vi "repeat cycle_exponential down.vi"(8 "error in (no error)":errorcluster caption="에러 입력(에러 없음)", 10 "waveform in":waveform(dbl), 11 "Waveform Obj 입력":refnum<class "Waveform Gen.lvclass">) -> (0 "error out":errorcluster caption="에러 출력", 2 "waveform out":waveform(dbl), 3 "Waveform Obj 출력":refnum<class "Waveform Gen.lvclass">)   [LabVIEW 2020, in "Waveform Gen.lvclass"]
uses:
  Waveform Gen.lvclass
  Waveform Gen.lvclass/Waveform Gen.ctl
  Accessors/Read cycle.vi
  <vilib>/Waveform/WDTOps.llb/WDT Append Waveforms DBL.vi
  <vilib>/Waveform/WDTOps.llb/WDT Number of Waveform Samples DBL.vi
  <vilib>/Waveform/WDTOps.llb/WDT Get Waveform Subset DBL.vi
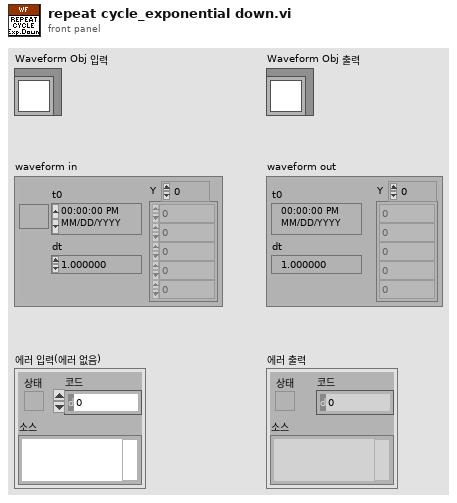
[diagram p1: front panel]
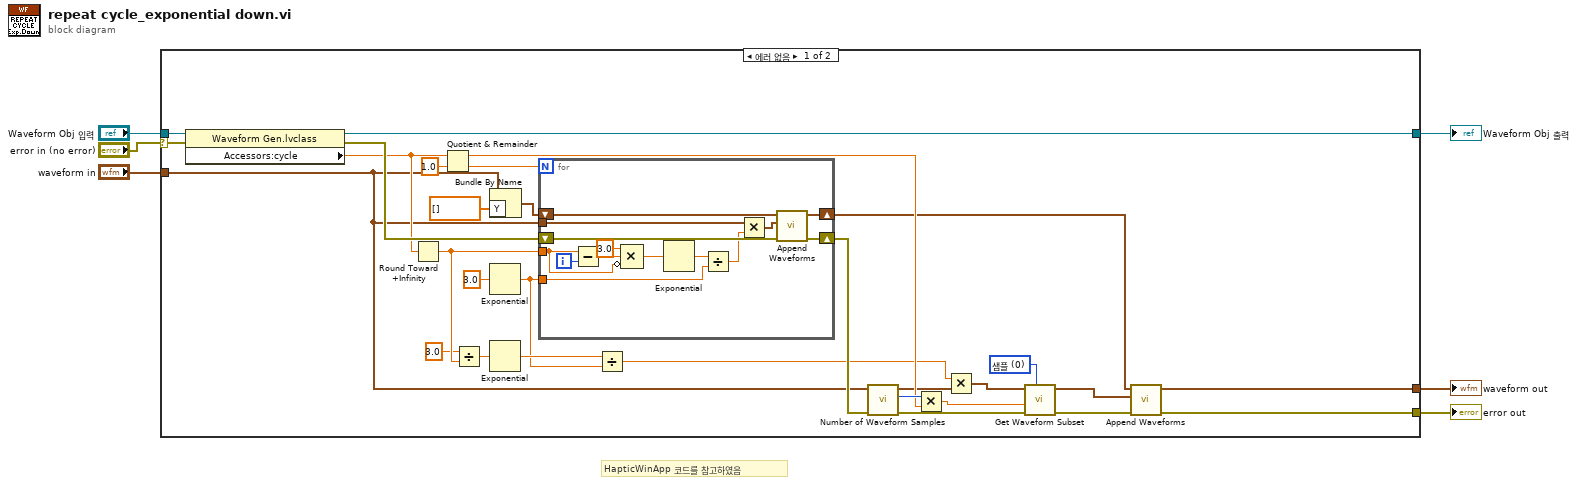
[diagram p0: block diagram]
diagram:
  # "HapticWinApp 코드를 참고하였음"
  n1 = case shown="에러 없음" "error in (no error)" {
    selector: "error in (no error)" -> [w34 w52]
    tunnel: [w8 w52] -> w3
    tunnel: "Waveform Obj 입력" -> [w36 w51]
    tunnel: [w9 w51] -> w4
    tunnel: "waveform in" -> [w10 _]
    tunnel: [w7 _] -> w1
    frame No Error {
      w23 = u16 0 items=["샘플", "상대 시간"] ("start/duration format")
      n2 = property class="Waveform Gen.lvclass"(reference=w36, error in=w34) -> (reference out=w9:refnum<class "Waveform Gen.lvclass">, error out=w27:errorcluster, "Accessors:cycle"=w22:dbl)
      n3 = Round Toward +Infinity(x=w22) -> (ceil(x): smallest int >= x=w19:dbl)
      n4 = Quotient & Remainder(x=w22, y=1.0) -> (x-y*floor(x/y)=w31:dbl, floor(x/y)=w33:dbl)
      n5 = Divide(x=3.0, y=w19) -> (x/y=w17:dbl)
      n6 = Bundle By Name(cluster=w10, "Y"=dbl[] []) -> (w11:waveform(dbl))
      n7 = Exponential(1:3.0 ("x")) -> (0:w15:dbl)
      n8 = Exponential(1:w17) -> (0:w16:dbl)
      n9 = for {
        N: w33 -> [_]
        shift-right: [w49] -> w13
        shift-left: w11 -> [w50]
        shift-right: [w47] -> w26
        shift-left: w27 -> [w48]
        tunnel: w10 -> [w46]
        tunnel: w19 -> [w41]
        tunnel: w15 -> [w38]
        i -> [w45]
        n10 = Subtract(x=w41, y=w45) -> (x-y=w43:dbl)
        n11 = Compound Arithmetic op=MULTIPLY(3.0 ("값"), w43, invert w41) -> (w40:dbl)
        n12 = Exponential(1:w40) -> (0:w39:dbl)
        n13 = Divide(x=w39, y=w38) -> (x/y=w37:dbl)
        n14 = Multiply(x=w46, y=w37) -> (x*y=w44:waveform(dbl))
        n15 = call-poly <vilib>:"Append Waveforms.vi"("error in (no error)"=w48, "waveform B"=w44, "waveform A"=w50) -> ("error out"=w47:errorcluster, "waveform out"=w49:waveform(dbl))  [unwired: 7 in]
      }
      n16 = Divide(x=w16, y=w15) -> (x/y=w14:dbl)
      n17 = call-poly <vilib>:"Number of Waveform Samples.vi"("error in (no error)"=w26, "waveform in"=w10) -> ("error out"=w29:errorcluster, "number of samples"=w32:i32, "waveform out"=w24:waveform(dbl))  [unwired: 7 in]
      n18 = Multiply(x=w32, y=w31) -> (x*y=w30:dbl)
      n19 = Multiply(x=w14, y=w24) -> (x*y=w21:waveform(dbl))
      n20 = call-poly <vilib>:"Get Waveform Subset.vi"("start/duration format"=w23, "error in (no error)"=w29, "duration"=w30, "waveform in"=w21) -> ("error out"=w25:errorcluster, "waveform out"=w28:waveform(dbl))  [unwired: 2 in, 2 out]
      n21 = call-poly <vilib>:"Append Waveforms.vi"("error in (no error)"=w25, "waveform B"=w28, "waveform A"=w13) -> ("error out"=w8:errorcluster, "waveform out"=w7:waveform(dbl))  [unwired: 7 in]
    }
    frame Error {
    }
  }
  "error out" <- w3
  "Waveform Obj 출력" <- w4
  "waveform out" <- w1
